vi "DAY 2 ,To View Excell Sheet (1).vi"() -> ()   [LabVIEW 2025]
uses:
  <vilib>/Utility/file.llb/Read Delimited Spreadsheet (string).vi
panel:
  in  "stop":bool
  in  "login":bool
  in  "Password":string
  in  "Username":string
  in  "file path (dialog if empty)":path
  out "all rows":string[][](array[string])
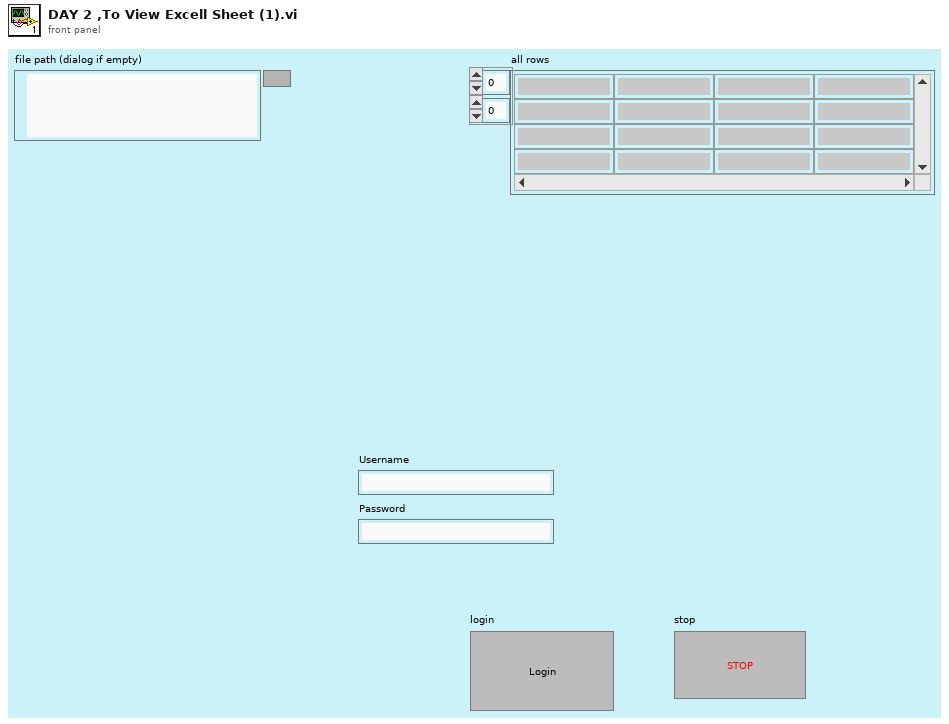
[diagram p1: front panel]
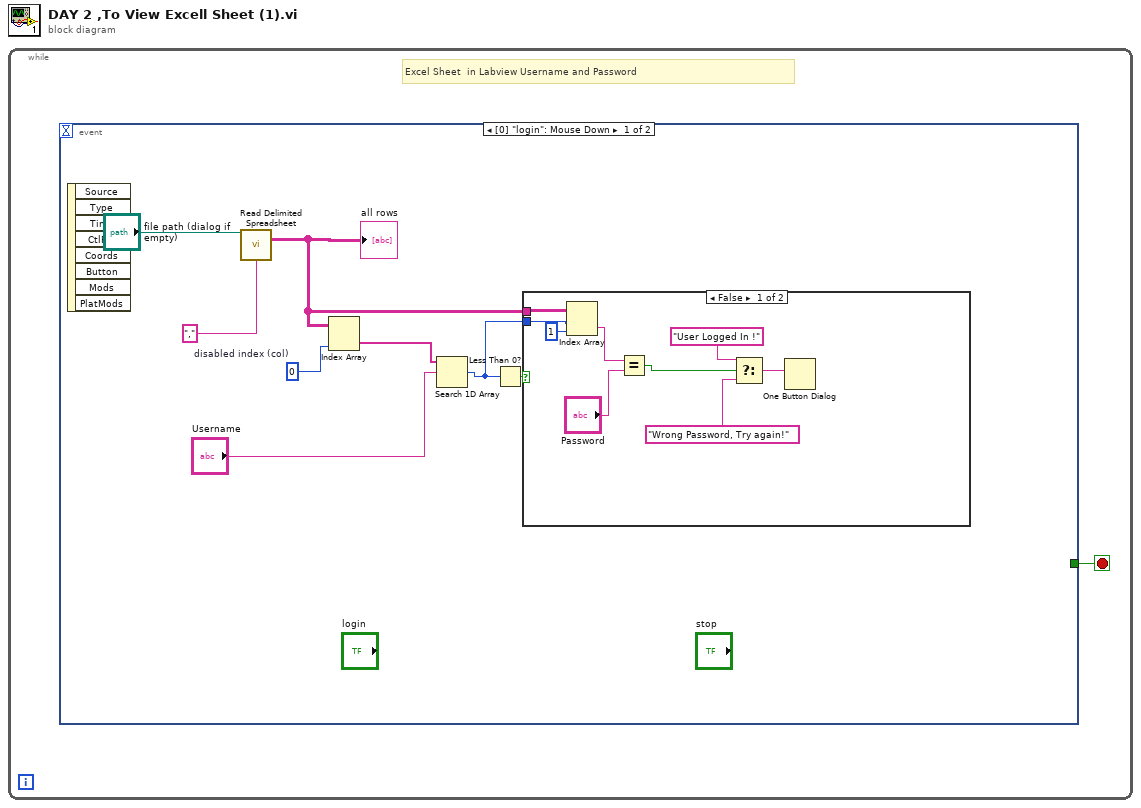
[diagram p0: block diagram]
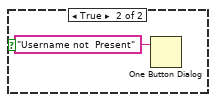
[diagram p2: hidden frame]
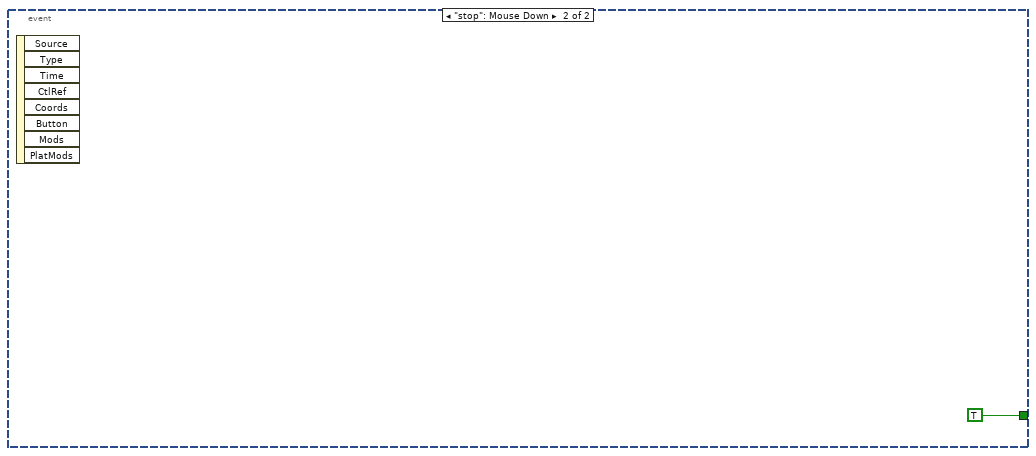
[diagram p3: hidden frame]
diagram:
  n1 = while {
    stop <- w1 stop-if-true
    # "Excel Sheet  in Labview Username and Password"
    n2 = event shown="[0] \"login\": Mouse Down" {
      selector: _ -> [_ _]
      dyn-events: _ -> [_ _]
      timeout: _ -> [_ _]
      tunnel: [_ TRUE] -> w1
      event "login": Mouse Down {
        w7 = 0  # disabled index (col)
        n3 = event-data() -> ()  [unwired: 1 in, 8 out]
        n4 = call-poly <vilib>:"Read Delimited Spreadsheet.vi"("file path (dialog if empty)"="file path (dialog if empty)", "delimiter (\\t)"="," ("delimiter (\\t)")) -> ("all rows"=w4:string[][])  [unwired: 8 in, 5 out]
        "all rows" <- w4
        n5 = Index Array(array=w4, index (col)=w7) -> (element=w6:string[])  [unwired: 1 in]
        n6 = Search 1D Array(1D array=w6, element="Username") -> (index of element=w3:i32)  [unwired: 1 in]
        n7 = Less Than 0?(x=w3) -> (x < 0?=w2:bool)
        n8 = case shown="False" w2 {
          tunnel: w4 -> [w18 _]
          tunnel: w3 -> [w16 _]
          frame False {
            n9 = Index Array(array=w18, index (row)=w16, index (col)=1 ("disabled index (col)")) -> (element=w14:string)
            n10 = Equal?(x=w14, y="Password") -> (x = y?=w13:bool)
            n11 = Select(t="User Logged In !", s=w13, f="Wrong Password, Try again!") -> (s? t:f=w10:string)
            n12 = One Button Dialog(message=w10) -> ()  [unwired: 1 in, 1 out]
          }
          frame True {
            n13 = One Button Dialog(message="Username not  Present") -> ()  [unwired: 1 in, 1 out]
          }
        }
      }
      event "stop": Mouse Down {
        n14 = event-data() -> ()  [unwired: 1 in, 8 out]
      }
    }
  }
